vi "AddToArraySmall_String.vi"(11 "String":string) -> (3 "output array":string[](array[string]))   [LabVIEW 2022 SP3]
doc: "Tager data som input og somætter det til et array."
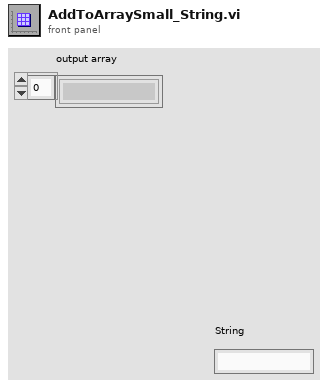
[diagram p1: front panel]
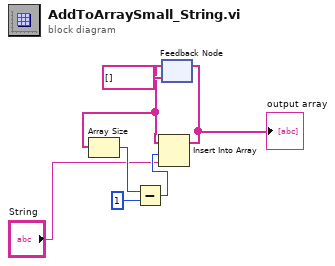
[diagram p0: block diagram]
diagram:
  n1 = feedback #1(string[] []) -> (w5:string[])
  n2 = Array Size(array=w5) -> (size(s)=w4:i32)
  n3 = Subtract(x=w4, y=1) -> (x-y=w2:i32)
  n4 = Insert Into Array(array=w5, index=w2, new element="String") -> (w6:string[])
  "output array" <- w6
  n5 = feedback-in #1(w6) -> ()
